vi "PrepInputFileForKepcoInput.vi"(8 "error in":errorcluster, 9 "Waveform List In":string[][](array[string]), 10 "Model In":string, 11 "VISA Session In":refnum<visa-resource-name>) -> (0 "error out":errorcluster, 1 "CurrentList":dbl[][](array[numeric]), 2 "Model Out":string, 3 "VISA Session Out":refnum<visa-resource-name>)   [LabVIEW 2013]
panel:
  out "Waveform Graph":T1(graph)={"Dwell (Sec)"=[0.0, 0.0005, 0.001, 0.0015], "Voltage Data"=[1.0, 2.0, 3.0]}
  out "number of points":i32=3 caption="Number of points"
  out "Total time":dbl=0.0015
  out "List not\nCorrected":bool
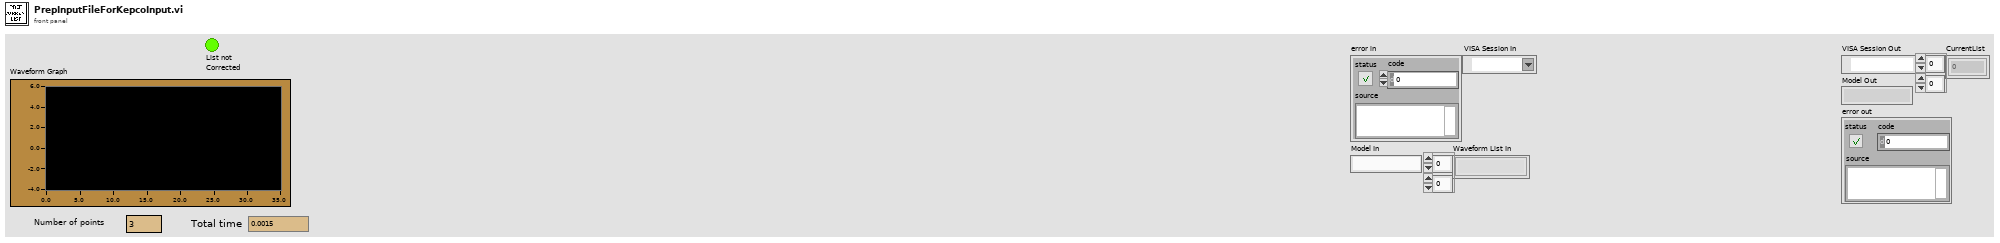
[diagram p1: front panel]
types:
  T1 = cluster{"Dwell (Sec)":dbl[], "Voltage Data":dbl[]}
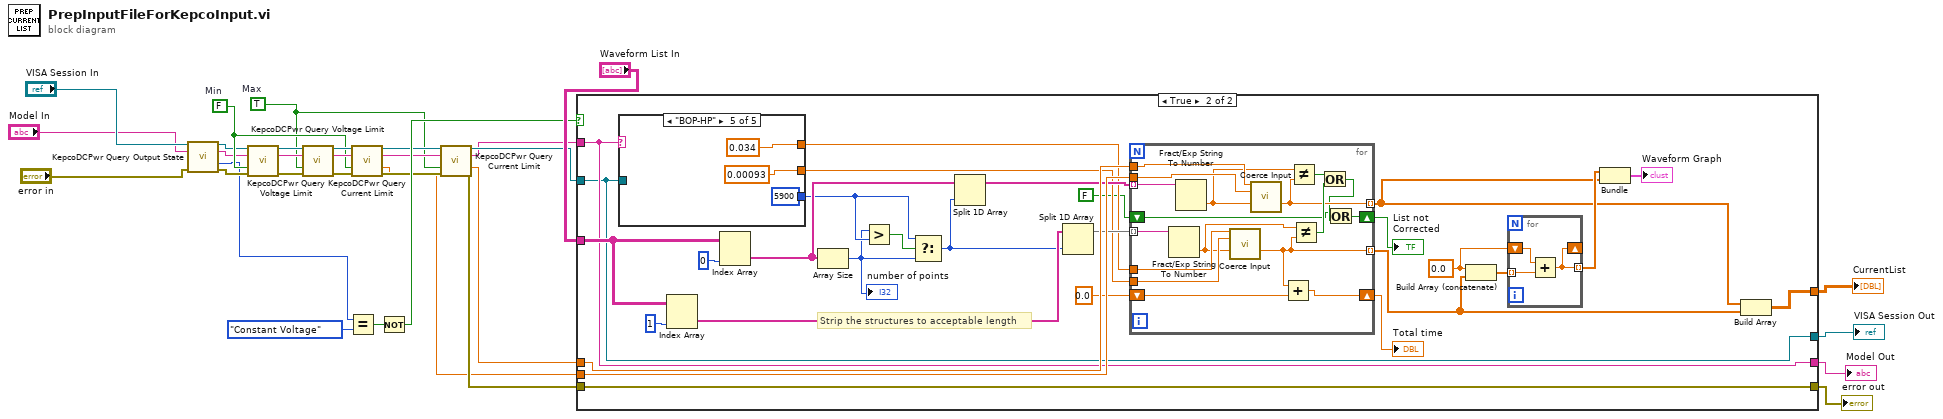
[diagram p0: block diagram]
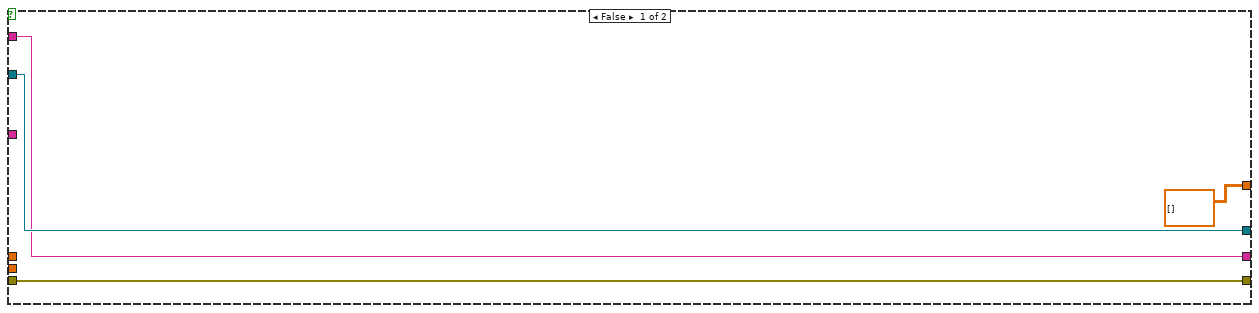
[diagram p2: hidden frame]
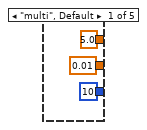
[diagram p3: hidden frame]
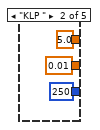
[diagram p4: hidden frame]
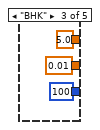
[diagram p5: hidden frame]
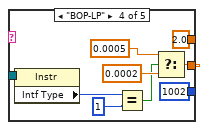
[diagram p6: hidden frame]
diagram:
  w14 = TRUE  # Max
  w15 = FALSE  # Min
  n1 = call "KepcoDCPwr Query Output State.vi"("VISA Session"="VISA Session In", "Model In"="Model In", "error in (no error)"="error in") -> ("VISA Session Out"=w13:refnum<visa-resource-name>, "Model Out"=w12:string, "Output state (Constant Voltage)"=w7:enum16{"Constatnt Voltage", "Constant Current"}, "error out"=w11:errorcluster)  [unwired: 5 in, 4 out]
  n2 = call "KepcoDCPwr Query Voltage Limit.vi"("VISA Session"=w13, "Model In"=w12, "Max Level (T),MIN LEVEL(F)"=w15, "error in (no error)"=w11) -> ("VISA Session Out"=w16:refnum<visa-resource-name>, "Model Out"=w23:string, "error out"=w24:errorcluster)  [unwired: 1 in, 8 out]
  n3 = call "KepcoDCPwr Query Voltage Limit.vi"("VISA Session"=w16, "Model In"=w23, "Max Level (T),MIN LEVEL(F)"=w14, "error in (no error)"=w24) -> ("VISA Session Out"=w17:refnum<visa-resource-name>, "Model Out"=w19:string, "error out"=w22:errorcluster)  [unwired: 1 in, 8 out]
  n4 = Equal?(x=w7, y=enum16{"Constant Voltage", "Constant Current"}."Constant Voltage" ("Output state (Constant Voltage)")) -> (x = y?=w26:bool)
  n5 = call "KepcoDCPwr Query Current Limit.vi"("VISA Session"=w17, "Model In"=w19, "Level"=w15, "error in (no error)"=w22) -> ("VISA Session Out"=w18:refnum<visa-resource-name>, "Model Out"=w20:string, "current limit"=w6:dbl, "error out"=w21:errorcluster)  [unwired: 1 in, 7 out]
  n6 = Not(x=w26) -> (.not. x?=w25:bool)
  n7 = call "KepcoDCPwr Query Current Limit.vi"("VISA Session"=w18, "Model In"=w20, "Level"=w14, "error in (no error)"=w21) -> ("VISA Session Out"=w10:refnum<visa-resource-name>, "Model Out"=w9:string, "current limit"=w5:dbl, "error out"=w8:errorcluster)  [unwired: 1 in, 7 out]
  n8 = case shown="True" w25 {
    tunnel: [dbl[][] [] w43] -> w4
    tunnel: w5 -> [_ w64]
    tunnel: w6 -> [_ w63]
    tunnel: "Waveform List In" -> [_ w51]
    tunnel: w10 -> [w35 w40]
    tunnel: w9 -> [w34 w48]
    tunnel: w8 -> [w33 w49]
    tunnel: [w33 w49] -> w2
    tunnel: [w35 w40] -> w3
    tunnel: [w34 w48] -> w1
    frame False {
    }
    frame True {
      w59 = 0.0
      # "Strip the structures to acceptable length"
      n9 = case shown="\"BOP-HP\"" w48 {
        tunnel: [5.0 5.0 5.0 2.0 0.034] -> w47
        tunnel: [0.01 0.01 0.01 w77 0.00093] -> w46
        tunnel: [10 250 100 1002 5900] -> w38
        tunnel: w40 -> [_ _ _ w80 _]
        frame "multi", Default {
        }
        frame "KLP " {
        }
        frame "BHK" {
        }
        frame "BOP-LP" {
          n10 = property class="Instr"(reference=w80) -> ("Intf Type"=w75:u16)  [unwired: 1 in, 2 out]
          n11 = Equal?(x=w75, y=u16 1 ("x")) -> (x = y?=w76:bool)
          n12 = Select(t=0.0005, s=w76, f=0.0002) -> (s? t:f=w77:dbl)
        }
        frame "BOP-HP" {
        }
      }
      n13 = Index Array(array=w51, index (col)=1) -> (element=w55:string[])  [unwired: 1 in]
      n14 = Index Array(array=w51, index (col)=0) -> (element=w50:string[])  [unwired: 1 in]
      n15 = Array Size(array=w50) -> (size(s)=w37:i32)
      "number of points" <- w37
      n16 = Greater?(x=w37, y=w38) -> (0:w39:bool)
      n17 = Select(t=w38, s=w39, f=w37) -> (s? t:f=w36:i32)
      n18 = Split 1D Array(array=w50, index=w36) -> (first subarray=w56:string[])  [unwired: 1 out]
      n19 = Split 1D Array(array=w55, index=w36) -> (first subarray=w54:string[])  [unwired: 1 out]
      n20 = for {
        tunnel: w56 -> [w102] mode=indexing
        tunnel: [w92] -> w44 mode=indexing
        tunnel: w54 -> [w101] mode=indexing
        tunnel: [w91] -> w45 mode=indexing
        tunnel: w64 -> [w93]
        tunnel: w63 -> [w100]
        shift-right: [w99] -> w52
        shift-left: 0.0 -> [w98]
        tunnel: w47 -> [w97]
        tunnel: w46 -> [w96]
        shift-right: [w86] -> w41
        shift-left: FALSE -> [w87]
        n21 = Fract/Exp String To Number(string=w101) -> (number=w89:dbl)  [unwired: 4 out]
        n22 = Fract/Exp String To Number(string=w102) -> (number=w90:dbl)  [unwired: 4 out]
        n23 = call "Coerce Input.vi"("Max"=w97, "Min"=w96, "Input"=w89) -> ("Output"=w91:dbl)  [unwired: 12 out]
        n24 = call "Coerce Input.vi"("Max"=w93, "Min"=w100, "Input"=w90) -> ("Output"=w92:dbl)  [unwired: 12 out]
        n25 = Add(x=w91, y=w98) -> (x+y=w99:dbl)
        n26 = Not Equal?(x=w90, y=w92) -> (x != y?=w95:bool)
        n27 = Not Equal?(x=w89, y=w91) -> (x != y?=w94:bool)
        n28 = Or(x=w95, y=w94) -> (x .or. y?=w88:bool)
        n29 = Or(x=w87, y=w88) -> (x .or. y?=w86:bool)
      }
      "Total time" <- w52
      "List not\nCorrected" <- w41
      n30 = Build Array (concatenate)(w59, w45) -> (w60:dbl[])
      n31 = for {
        tunnel: w60 -> [w105] mode=indexing
        shift-right: [w103] -> _
        shift-left: w59 -> [w104]
        tunnel: [w103] -> w61 mode=indexing
        n32 = Add(x=w104, y=w105) -> (x+y=w103:dbl)
      }
      n33 = Bundle(w61, w44) -> (→"Waveform Graph":cluster{dbl[], dbl[]})  [unwired: 1 out]
      n34 = Build Array(w44, w45) -> (w43:dbl[][])
    }
  }
  "VISA Session Out" <- w3
  "Model Out" <- w1
  "error out" <- w2
  "CurrentList" <- w4
